vi "__uintMaxMin.vi"(10 "Uint2 in":u8[](array[numeric])=[0], 11 "Uint1 in":u8[](array[numeric])=[0]) -> (0 "Timing":u32, 2 "Min":u8[](array[numeric]), 3 "Max":u8[](array[numeric]))   [LabVIEW 2011, in "UintClass.lvclass"]
uses:
  UintClass.lvclass
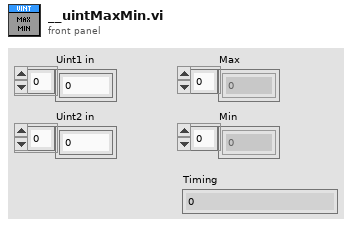
[diagram p1: front panel]
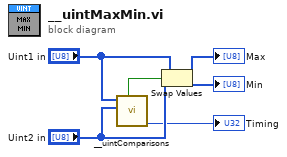
[diagram p0: block diagram]
diagram:
  n1 = call "__uintComparisons.vi"("Uint2 in"="Uint2 in", "Uint1 in"="Uint1 in") -> ("Timing comparison"=→"Timing":u32, "Uint1 < Uint2"=w2:bool)  [unwired: 3 in, 5 out]
  n2 = Swap Values(12:"Uint1 in", 13:w2, 14:"Uint2 in") -> (1:→"Max":u8[], 3:→"Min":u8[])
